vi "Fault States to Word.vi"(11 "Fault States":T1[](array[typedef])) -> (3 "Fault Word":u16)   [LabVIEW 2014, in "SLSC configuration Shared.lvlib"]
doc: "Converts four faults to a fault word."
uses:
  SLSC configuration Shared.lvlib
  Fault State.ctl
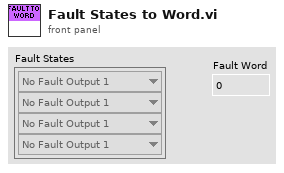
[diagram p1: front panel]
types:
  T1 = typedef "SLSC configuration Shared.lvlib/Fault State.ctl" = enum8{"No Fault Output 1", "Open Circuit 100 Hz", "Ground 100 Hz", "Open Circuit", "Ground", "Fail Rail 1", "Fail Rail 2", "No Fault Output 2"}
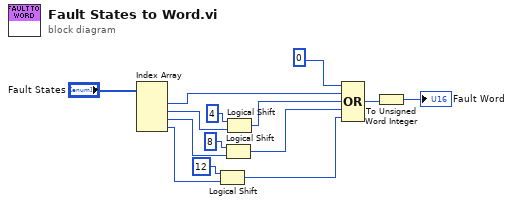
[diagram p0: block diagram]
diagram:
  n1 = Index Array(array="Fault States") -> (element #1=w9:T1, element #2=w3:T1, element #3=w4:T1, element #4=w5:T1)  [unwired: 4 in]
  n2 = Logical Shift(y=u16 12, x=w5) -> (x << y=w12:u32)
  n3 = Logical Shift(y=u16 8, x=w4) -> (x << y=w11:u32)
  n4 = Logical Shift(y=u16 4, x=w3) -> (x << y=w10:u32)
  n5 = Compound Arithmetic op=OR(u16 0 ("value"), w9, w10, w11, w12) -> (w13:u32)
  n6 = To Unsigned Word Integer(number=w13) -> (unsigned 16bit integer=→"Fault Word":u16)
